vi "PixyCam_Example.vi"() -> ()   [LabVIEW 2016]
uses:
  Private/PixyCam_CommMode.ctl
  <vilib>/Rock Robotics/SystemInterfaces/spilib/spi_bus.ctl
  PixyCam_LabVIEW.lvlib
  <vilib>/vision/NI_Vision_Development_Module.lvlib
panel:
  in  "Color Pixel Value":u32(colorbox)=15775779
  in  "Brightness":u8=40
  out "Targets":T1(plugin-control)
  in  "stop":bool
  in  "SPI Bus":T2
  in  "Communication Mode":T3
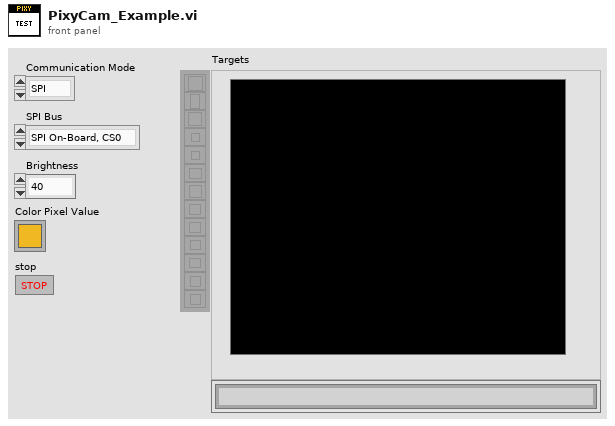
[diagram p1: front panel]
types:
  T1 = typedef "IMAQ Image.ctl" = refnum<image>
  T2 = typedef "spi_bus.ctl" = enum16{"SPI On-Board, CS0", "SPI On-Board, CS1", "SPI On-Board, CS2", "SPI On-Board, CS3", "SPI MXP", "Invalid"}
  T3 = typedef "PixyCam_LabVIEW.lvlib/PixyCam_CommMode.ctl" = enum16{"SPI", "I2C", "UART", "Analog", "Digital"}
  T4 = typedef "Image Type" = u32
  T5 = typedef "PixyCam_LabVIEW.lvlib/PixyCam_DevRef.ctl" = cluster{"PixyCamDevRef_SPI":T6, "Communication Mode":T3, "Error":errorcluster}
  T6 = typedef "PixyCam_LabVIEW.lvlib/PixyCam_SPI_DevRef.ctl" = cluster{"SPIDevRef":T7, "Output Queue":refnum<queue>}
  T7 = typedef "WPI_SPIDevRef.ctl" = cluster{"DevStatus":errorcluster, "Handle":i32, "SPI Bus":T2}
  T8 = cluster{"Left":i32, "Top":i32, "Right":i32, "Bottom":i32}
  T9 = typedef "PixyCam_LabVIEW.lvlib/PixyCam_TargetData.ctl" = cluster{"Target Type":u16, "Checksum":u16, "Signature Number":u16, "X Center":u16, "Y Center":u16, "Width":u16, "Height":u16, "Angle":u16}
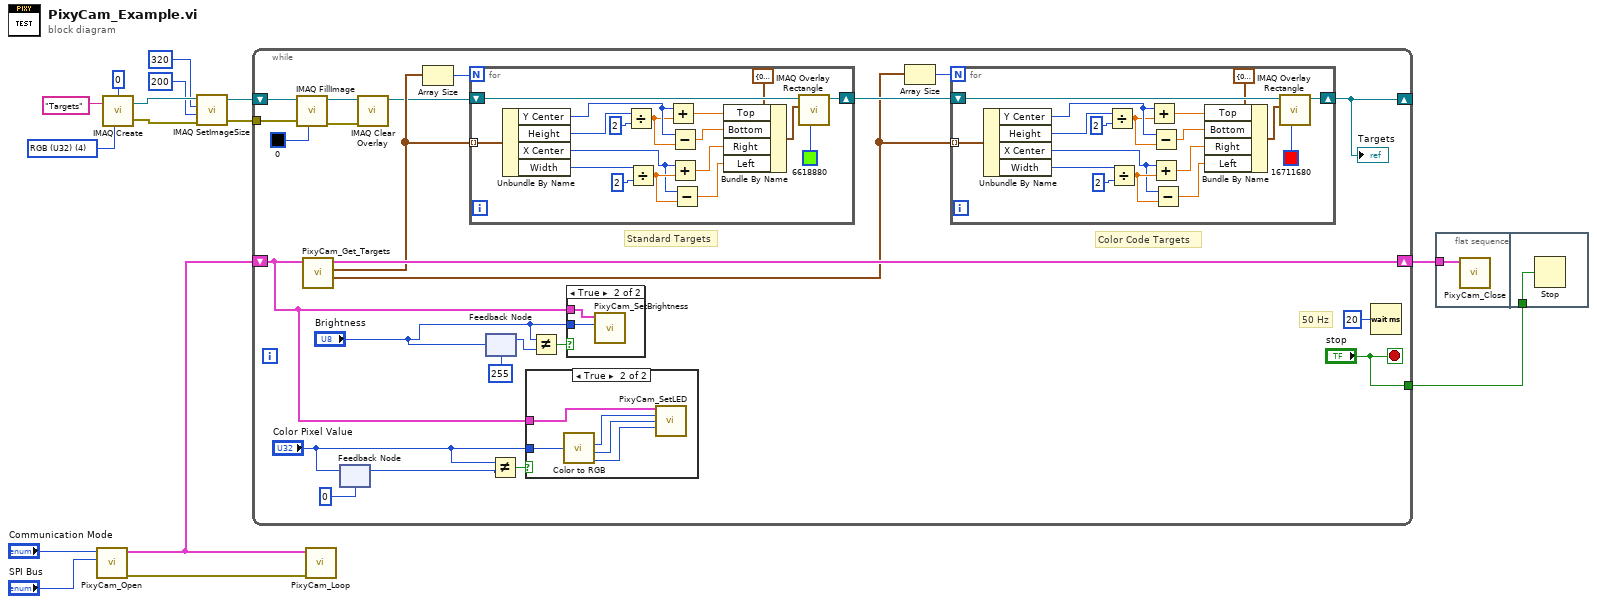
[diagram p0: block diagram]
diagram:
  w10 = T4 4 items=["Grayscale (U8)", "Grayscale (I16)", "Grayscale (SGL)", "Complex (CSG)", "RGB (U32)", "HSL (U32)", "RGB (U64)", "Grayscale (U16)"] ("Image Type")
  n1 = call "PixyCam_Open.vi"("SPI Bus"="SPI Bus", "Communication Mode"="Communication Mode") -> ("error out"=w11:errorcluster, "output cluster"=w13:T5)  [unwired: 4 in]
  n2 = call "IMAQ Create"("Border Size"=0, "Image Name"="Targets", "Image Type"=w10) -> ("New Image"=w6:T1, "error out"=w7:errorcluster)  [unwired: 2 in]
  n3 = call "IMAQ SetImageSize"("error in (no error)"=w7, "Y Resolution"=200, "X Resolution"=320, "Image"=w6) -> ("error out"=w2:errorcluster, "Image Out"=w3:T1)  [unwired: 1 in]
  n4 = while {
    shift-right: [w34] -> _
    shift-left: w3 -> [w38]
    shift-right: [w36] -> w12
    shift-left: w13 -> [w22]
    tunnel: w2 -> [w27]
    tunnel: ["stop"] -> w1
    stop <- "stop" stop-if-true
    # "50 Hz"
    # "Color Code Targets"
    # "Standard Targets"
    n5 = call "IMAQ FillImage"("Color Pixel Value"=u32 0, "error in (no error)"=w27, "Image"=w38) -> ("error out"=w32:errorcluster, "Image Out"=w33:T1)  [unwired: 7 in]
    n6 = call "PixyCam_Get_Targets.vi"("PixyCamDevRef"=w22) -> ("ColorCodeTargets Out"=w30:T9[], "StandardTargets Out"=w29:T9[], "PixyCamDevRef Out"=w36:T5)  [unwired: 4 in]
    n7 = feedback #1(u32 0 ("Color Pixel Value")) -> (w21:u32)
    n8 = feedback-in #1("Color Pixel Value") -> ()
    n9 = call "IMAQ Clear Overlay"("error in (no error)"=w32, "Image"=w33) -> ("Image Out"=w28:T1)  [unwired: 8 in, 1 out]
    n10 = Array Size(array=w29) -> (size(s)=w17:i32)
    n11 = for {
      N: w17 -> [_]
      shift-right: [w80] -> w35
      shift-left: w28 -> [w82]
      tunnel: w29 -> [w65] mode=indexing
      n12 = Unbundle By Name(w65) -> ("Y Center"=w75:u16, "Height"=w77:u16, "X Center"=w69:u16, "Width"=w68:u16)
      n13 = Divide(x=w77, y=u16 2) -> (x/y=w74:dbl)
      n14 = Divide(x=w68, y=u16 2) -> (x/y=w71:dbl)
      n15 = Add(x=w75, y=w74) -> (x+y=w72:dbl)
      n16 = Subtract(x=w75, y=w74) -> (x-y=w73:dbl)
      n17 = Add(x=w69, y=w71) -> (x+y=w67:dbl)
      n18 = Subtract(x=w69, y=w71) -> (x-y=w66:dbl)
      n19 = Bundle By Name(cluster=T8 {"Left"=0, "Top"=0, "Right"=0, "Bottom"=0} ("Rectangle"), "Top"=w72, "Bottom"=w73, "Right"=w67, "Left"=w66) -> (w78:T8)
      n20 = call "IMAQ Overlay Rectangle"("Color"=u32 6618880, "Rectangle"=w78, "Image"=w82) -> ("Image Out"=w80:T1)  [unwired: 7 in, 1 out]
    }
    n21 = feedback-in #2("Brightness") -> ()
    n22 = feedback #2(u8 255 ("Brightness")) -> (w24:u8)
    n23 = Not Equal?(x="Color Pixel Value", y=w21) -> (x != y?=w19:bool)
    n24 = case shown="True" w19 {
      tunnel: w22 -> [_ w44]
      tunnel: "Color Pixel Value" -> [_ w43]
      frame False {
      }
      frame True {
        n25 = call <vilib>:"Color to RGB.vi"("Color"=w43) -> ("R"=w42:u8, "G"=w41:u8, "B"=w40:u8)  [unwired: 1 out]
        n26 = call "PixyCam_SetLED.vi"("PixyCamDevRef"=w44, "Red"=w42, "Green"=w41, "Blue"=w40) -> ()  [unwired: 10 in, 2 out]
      }
    }
    n27 = Not Equal?(x="Brightness", y=w24) -> (x != y?=w25:bool)
    n28 = case shown="True" w25 {
      tunnel: w22 -> [_ w46]
      tunnel: "Brightness" -> [_ w45]
      frame False {
      }
      frame True {
        n29 = call "PixyCam_SetBrightness.vi"("Brightness"=w45, "PixyCamDevRef"=w46) -> ()  [unwired: 4 in, 2 out]
      }
    }
    n30 = Array Size(array=w30) -> (size(s)=w31:i32)
    n31 = for {
      N: w31 -> [_]
      tunnel: w30 -> [w61] mode=indexing
      shift-right: [w62] -> w34
      shift-left: w35 -> [w64]
      n32 = Unbundle By Name(w61) -> ("Y Center"=w56:u16, "Height"=w58:u16, "X Center"=w50:u16, "Width"=w49:u16)
      n33 = Divide(x=w58, y=u16 2) -> (x/y=w55:dbl)
      n34 = Divide(x=w49, y=u16 2) -> (x/y=w52:dbl)
      n35 = Add(x=w56, y=w55) -> (x+y=w53:dbl)
      n36 = Subtract(x=w56, y=w55) -> (x-y=w54:dbl)
      n37 = Add(x=w50, y=w52) -> (x+y=w48:dbl)
      n38 = Subtract(x=w50, y=w52) -> (x-y=w47:dbl)
      n39 = Bundle By Name(cluster=T8 {"Left"=0, "Top"=0, "Right"=0, "Bottom"=0} ("Rectangle"), "Top"=w53, "Bottom"=w54, "Right"=w48, "Left"=w47) -> (w59:T8)
      n40 = call "IMAQ Overlay Rectangle"("Color"=u32 16711680, "Rectangle"=w59, "Image"=w64) -> ("Image Out"=w62:T1)  [unwired: 7 in, 1 out]
    }
    "Targets" <- w34
    n41 = Wait (ms)(milliseconds to wait=u32 20) -> ()  [unwired: 1 out]
  }
  n42 = call "PixyCam_Loop.vi"("error in"=w11, "PixyCamDevRef"=w13) -> ()  [unwired: 4 in, 2 out]
  n43 = flat-sequence {
    tunnel: w12 -> [w83]
    tunnel: w1 -> [w84]
    frame #0 {
      n44 = call "PixyCam_Close.vi"("PixyCamDevRef"=w83) -> ()  [unwired: 6 in, 1 out]
    }
    frame #1 {
      n45 = Stop(stop? (T)=w84) -> ()
    }
  }
